vi "mid_str.vi"(4 "String":string="f(e)") -> (1 "mid substring":string)   [LabVIEW 2010]
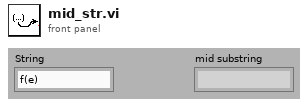
[diagram p1: front panel]
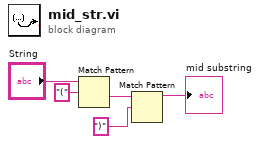
[diagram p0: block diagram]
diagram:
  n1 = Match Pattern(string="String", regular expression="(") -> (after substring=w3:string)  [unwired: 1 in, 3 out]
  n2 = Match Pattern(string=w3, regular expression=")") -> (before substring=→"mid substring":string)  [unwired: 1 in, 3 out]
